vi "5.vi"(11 "文字列入力":string) -> (3 "文字列出力":string)   [LabVIEW 2019]
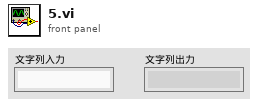
[diagram p1: front panel]
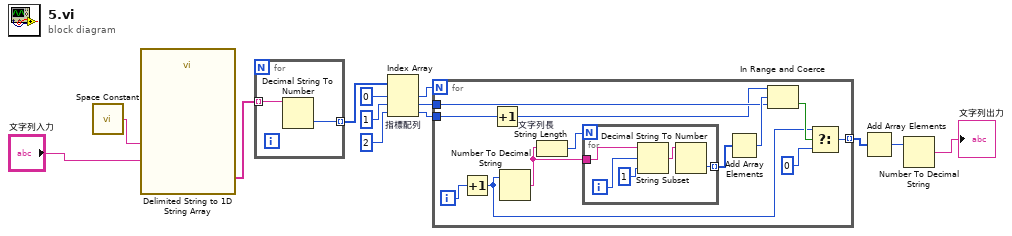
[diagram p0: block diagram]
diagram:
  n1 = call <vilib>:"Space Constant.vi"() -> ("String"=w1:string)
  n2 = call <vilib>:"Delimited String to 1D String Array.vi"("delimiter"=w1, "delimited string"="文字列入力") -> ("string array"=w3:string[])  [unwired: 9 in]
  n3 = for {
    tunnel: w3 -> [w15] mode=indexing
    tunnel: [w14] -> w6 mode=indexing
    n4 = Decimal String To Number(string=w15) -> (number=w14:i32)  [unwired: 2 in, 1 out]
  }
  n5 = Index Array "指標配列"(array=w6, index #1=0, index #2=1, index #3=2) -> (element #1=w8:i32, element #2=w9:i32, element #3=w10:i32)
  n6 = for {
    N: w8 -> [_]
    tunnel: w9 -> [w23]
    tunnel: w10 -> [w22]
    tunnel: [w19] -> w11 mode=indexing
    i -> [w18]
    n7 = Increment(x=w18) -> (x+1=w17:i32)
    n8 = Increment(x=w22) -> (x+1=w16:i32)
    n9 = Number To Decimal String(number=w17) -> (decimal integer string=w26:string)  [unwired: 1 in]
    n10 = String Length "文字列長"(string=w26) -> (length=w27:i32)
    n11 = for {
      N: w27 -> [_]
      tunnel: w26 -> [w32]
      tunnel: [w28] -> w25 mode=indexing
      i -> [w30]
      n12 = String Subset(string=w32, offset (0)=w30, length (rest)=1 ("長さ (残り)")) -> (substring=w29:string)
      n13 = Decimal String To Number(string=w29) -> (number=w28:i32)  [unwired: 2 in, 1 out]
    }
    n14 = Add Array Elements(numeric array=w25) -> (sum=w24:i32)
    n15 = In Range and Coerce(upper limit=w16, x=w24, lower limit=w23) -> (In Range?=w21:bool)  [unwired: 1 out]
    n16 = Select(t=w17, s=w21, f=0) -> (s? t:f=w19:i32)
  }
  n17 = Add Array Elements(numeric array=w11) -> (sum=w12:i32)
  n18 = Number To Decimal String(number=w12) -> (decimal integer string=→"文字列出力":string)  [unwired: 1 in]
